vi "FGV ARN Test.vi"(7 "abgebrochen":bool, 10 "Aktion":T1=enum."init") -> (0 "Tabelle Wertänderung":bool, 1 "Fertig":bool, 2 "Aktion":T1=enum."init", 3 "Status":string)   [LabVIEW 2020, in "EPA 1065.lvlib" / "ARN Test 1065-305.lvlib"]
uses:
  ARN Test 1065-305.lvlib
  Aktion FGV ARN Test.ctl
  Aktion FGV ARN Daten.ctl
  Seiten/FT-IR/FGV FT-IR Aktionen.ctl
  Sprachverwaltung/FGV Aktion Tabelle zerlegen.ctl
  Seiten/CalGas Aufschaltung/FGV CalGas Aktionen.ctl
  Aktion FGV Graphen Daten.ctl
  Funktionstasten/Zustaende.ctl
  Funktionstasten/Funktionstasten-Aktion.ctl
  Seiten/CalGas Aufschaltung/Auswahl Aufschaltpunkt.ctl
  PNS/Aktionen FGV Grenzwerte.ctl
  Messdaten/Aktionen FGV Messdaten.ctl
  Messdaten/Gewichtung (Stichprobe).ctl
  Aktion FGV ARN Protokoll.ctl
  Funktionstasten/Funktionstasten.lvlib
  Messdaten/Messdaten.lvlib
  Seiten/FT-IR/FT-IR.lvlib
  Sprachverwaltung/Sprachverwaltung.lvlib
  Seiten/CalGas Aufschaltung/CalGas Aufschaltung.lvlib
  PNS/PNS.lvlib
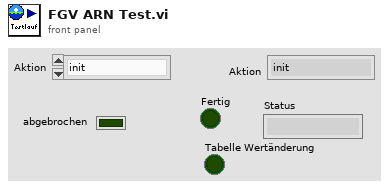
[diagram p1: front panel]
types:
  T1 = typedef "EPA 1065.lvlib/ARN Test 1065-305.lvlib/Aktion FGV ARN Test.ctl" = enum16{"leerlauf", "init", "lesen", "CG aufschalten", "Aufschaltzeit abwarten", "aufzeichnen vorbereiten", "aufzeichnen", "berechnen", "auswerten", "fertig", "0-Gas aufschalten", "0-Gas abwarten"}
  T2 = typedef "EPA 1065.lvlib/ARN Test 1065-305.lvlib/Aktion FGV Graphen Daten.ctl" = enum16{"init", "lesen", "Daten schreiben"}
  T3 = typedef "CalGas Aufschaltung.lvlib/FGV CalGas Aktionen.ctl" = enum16{"lesen", "Analysator Auswahl", "Def.CalGas", "Aufschaltung CalGas", "laden", "speichern", "KAL extrahieren"}
  T4 = enum16{"init", "lesen", "ARN Test aktiv", "ARN Test inaktiv"}
  T5 = typedef "Sprachverwaltung.lvlib/FGV Aktion Tabelle zerlegen.ctl" = enum16{"laden", "vereinzeln", "speichern"}
  T6 = typedef "EPA 1065.lvlib/ARN Test 1065-305.lvlib/Aktion FGV ARN Daten.ctl" = enum16{"Lesen", "laden", "speichern", "ARN Daten", "Rohdaten", "Rohdaten löschen", "Zeitstempel", "SNR Ergebnis"}
  T7 = typedef "FT-IR.lvlib/FGV FT-IR Aktionen.ctl" = enum16{"lesen", "NOG setzen", "NOS setzen", "Initialisieren", "speichern", "ALLES setzen", "FT-IR Spektrum loggen", "Komm Stoppen", "Spektrum LogKonfig"}
  T8 = typedef "Messdaten.lvlib/Aktionen FGV Messdaten.ctl" = enum16{"lesen", "schreiben", "löschen", "Mittelwerte", "Komponente"}
  T9 = typedef "CalGas Aufschaltung.lvlib/Auswahl Aufschaltpunkt.ctl" = enum16{"über Filterblock", "Analysator direkt", "über PNS", "Entnahme", "Gasdivider"}
  T10 = typedef "Funktionstasten.lvlib/Funktionstasten-Aktion.ctl" = enum16{"Initialisieren", "Zustand setzen", "Taste gedrückt", "Fehler speichern", "Lesen", "Manuell", "Remote", "Bitparallel", "Samplepoint", "Zeit Prüfen", "reset Umschalten"}
  T11 = typedef "Funktionstasten.lvlib/Zustaende.ctl" = enum16{"Standby", "Pause", "Eco", "Messen", "Kalibrieren", "Spülen Filter", "Spülen Leitung", "Umgebungsluft", "0-Gas", "Cal-Gas", "CG zu PNS", "-------------", "Init 1", "Init 2", "Init 3", "Init 4", "Messen vorbereiten", "Messen durchführen", "Exit"}
  T12 = typedef "PNS.lvlib/Aktionen FGV Grenzwerte.ctl" = enum16{"lesen", "Grenzw. schreiben", "Anweisungscode", "IP-Adresse", "laden", "speichern", "Anweisungscode vorgeben"}
  T13 = typedef "EPA 1065.lvlib/ARN Test 1065-305.lvlib/Aktion FGV ARN Protokoll.ctl" = enum16{"lesen", "Tab. schreiben", "Protokoll ausw.", "Protokoll speichern", "Textdatei speichern"}
  T14 = typedef "Messdaten.lvlib/Gewichtung (Stichprobe).ctl" = enum16{"Sample", "Population"}
  T15 = typedef "EPA 1065.lvlib/ARN Test 1065-305.lvlib/Allgemeine Einstellungen.ctl" = cluster{"Bearbeiter:":string, "Analysator":T16, "Komponente:":u16, "Gasflaschen Nr.:":string, "Accuracy":dbl, "Sollwert":dbl, "Modus":T17, "Pfad:":path, "Textname:":string, "CG Aufschaltzeit:":dbl, "Einheit":string, "N2 Aufschaltzeit:":dbl, "Gasflasche":T18, "Konfig Gasflasche":T19}
  T16 = typedef "System Einstellungen V2.lvlib/Analysatoren.ctl" = string
  T17 = typedef "EPA 1065.lvlib/T90 Test 1065-308.lvlib/Modus.ctl" = u16
  T18 = typedef "System Einstellungen V2.lvlib/Gasflasche Auswahl.ctl" = u16
  T19 = typedef "System Einstellungen V2.lvlib/Konfig Gasflasche.ctl" = bool
  T20 = typedef "CalGas Aufschaltung.lvlib/Aufschaltung CalGas.ctl" = cluster{"Kalibriergas":T21, "Aufschaltpunkt":T9, "Analysator":T22}
  T21 = typedef "Auswahlfeld.ctl" = u16
  T22 = typedef "CalGas Aufschaltung.lvlib/Auswahl Analysator.ctl" = enum16{"FT-IR", "FID", "PMA", "PMA/FID/FT-IR"}
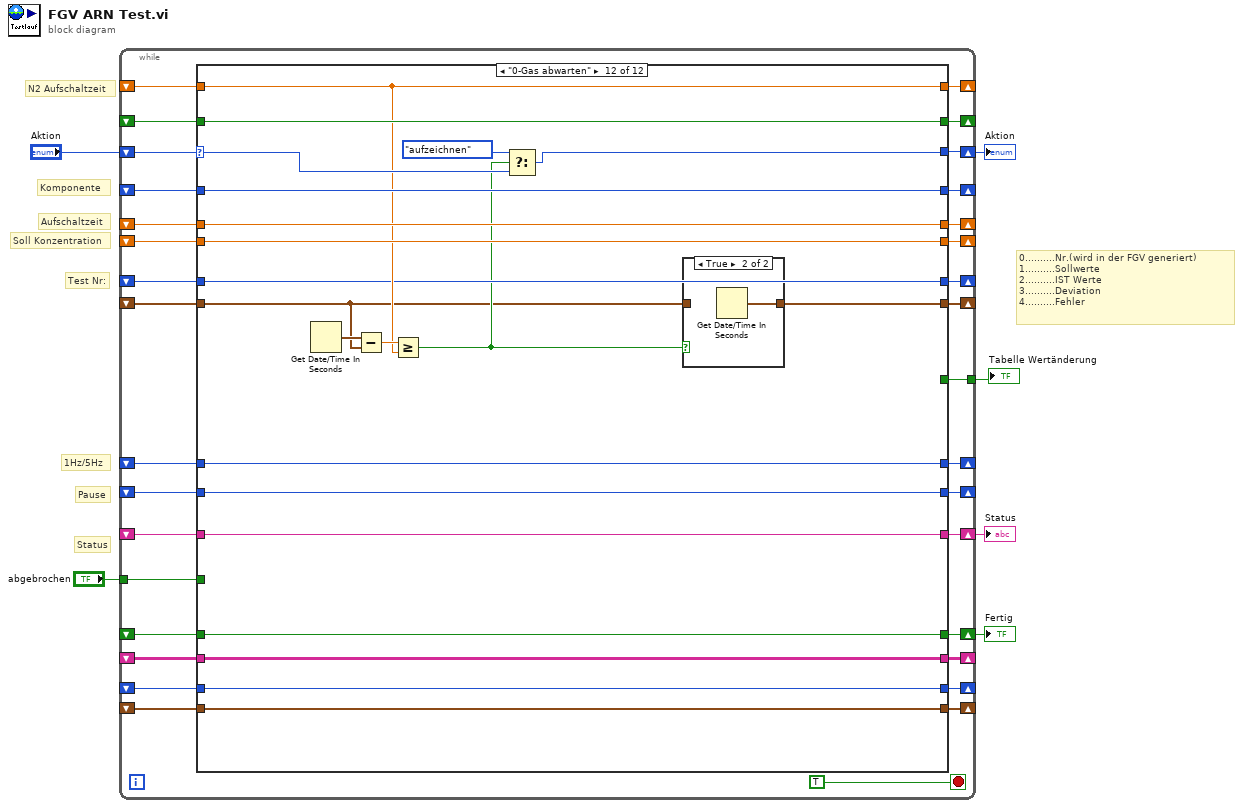
[diagram p0: block diagram]
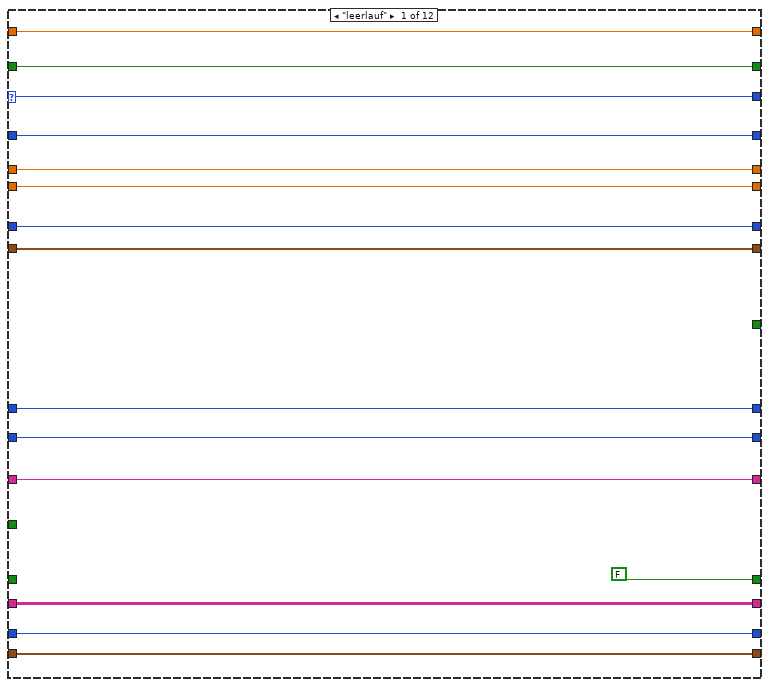
[diagram p2: hidden frame]
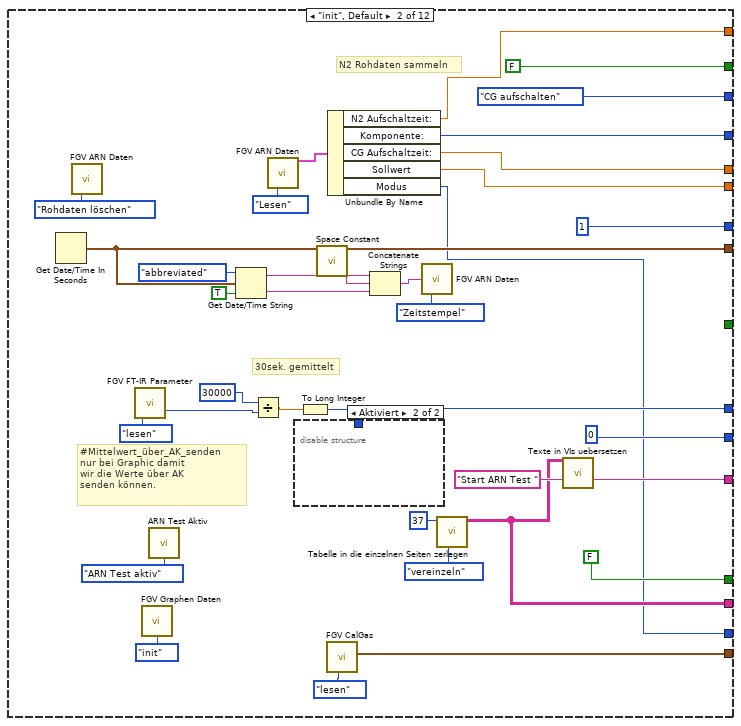
[diagram p3: hidden frame]
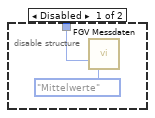
[diagram p4: hidden frame]
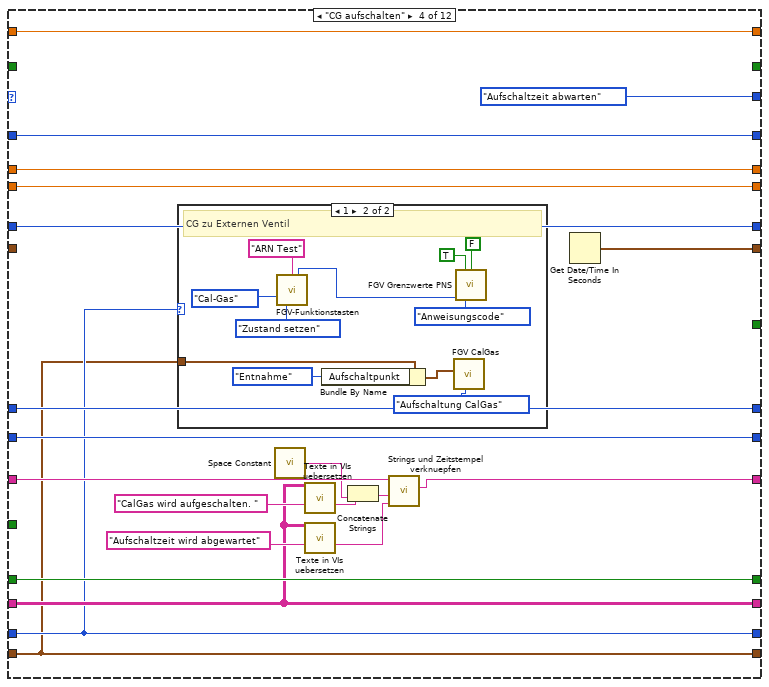
[diagram p6: hidden frame]
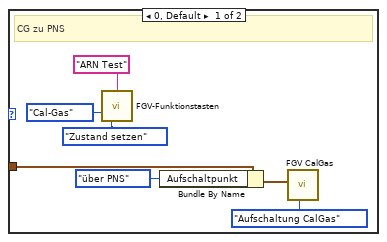
[diagram p7: hidden frame]
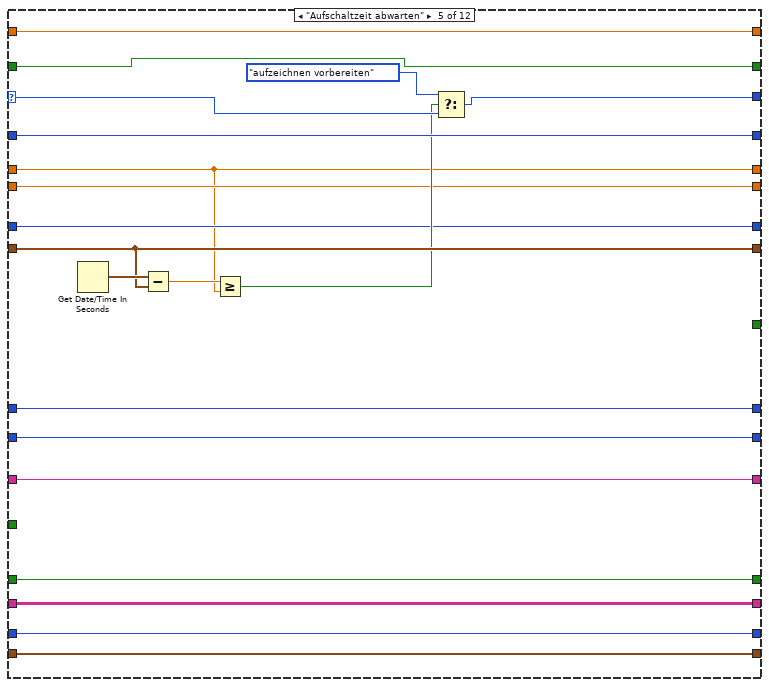
[diagram p8: hidden frame]
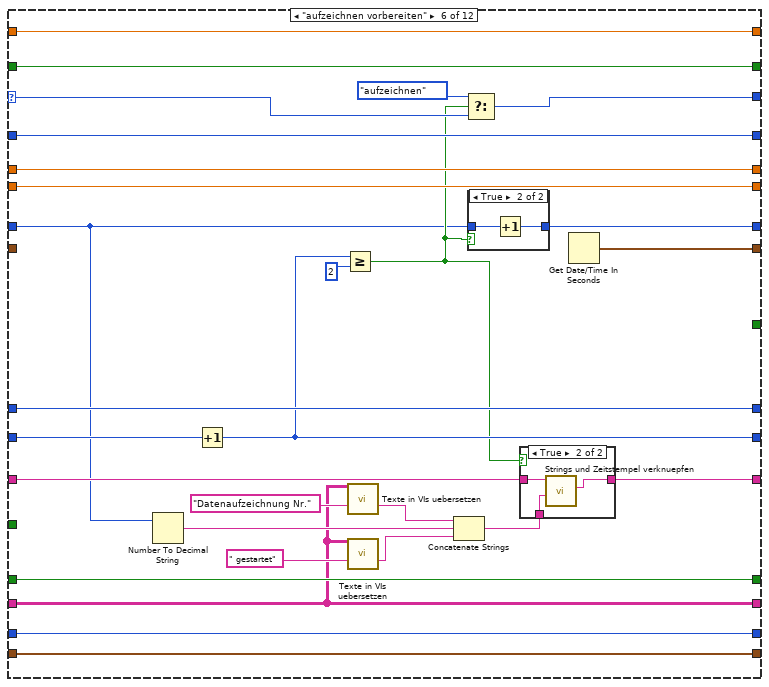
[diagram p9: hidden frame]
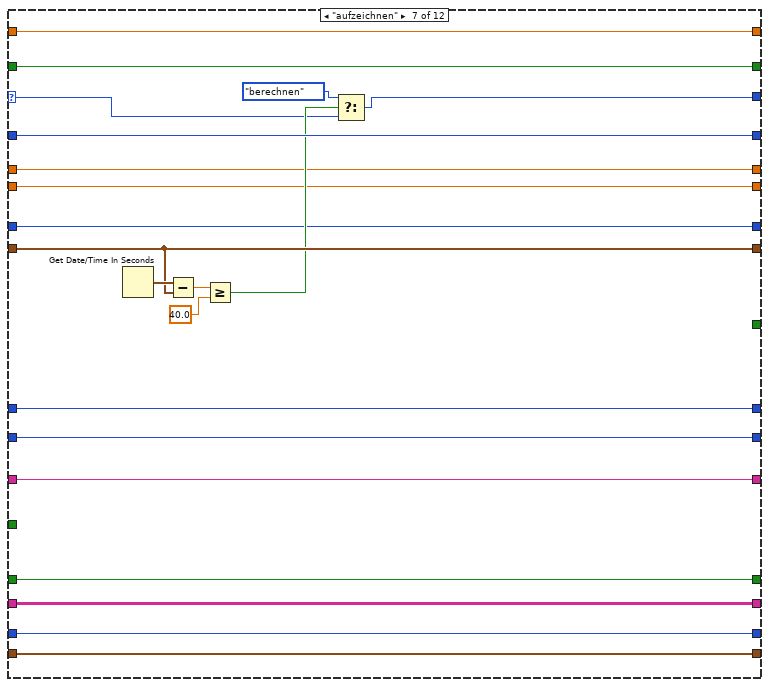
[diagram p12: hidden frame]
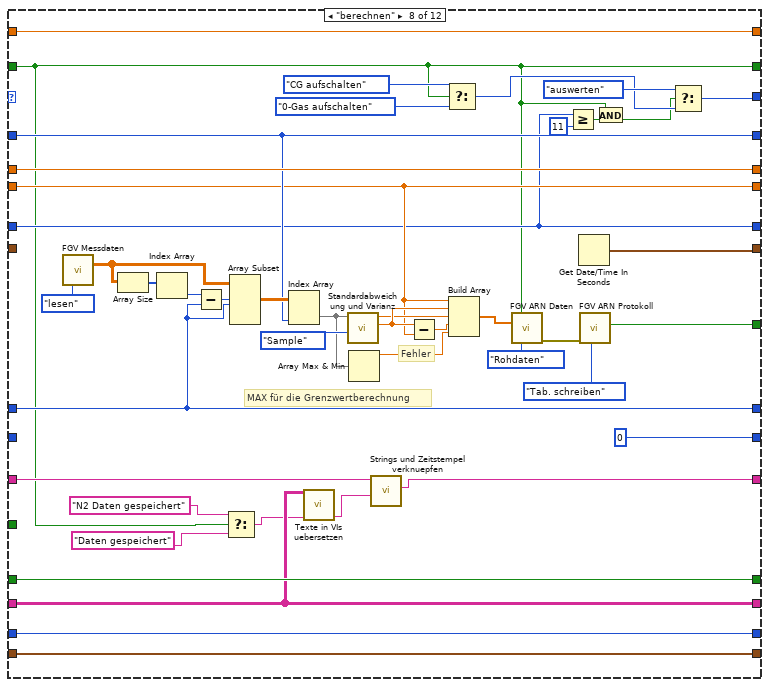
[diagram p13: hidden frame]
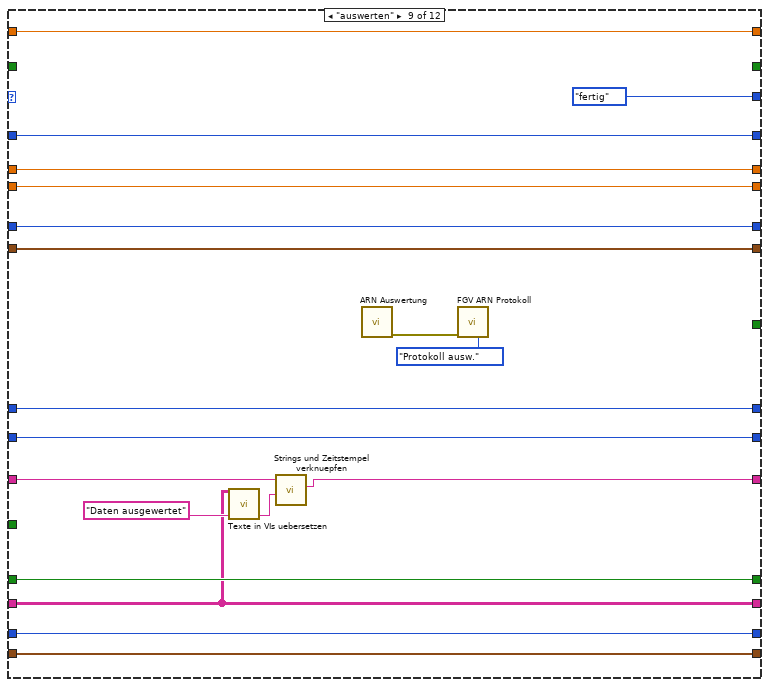
[diagram p14: hidden frame]
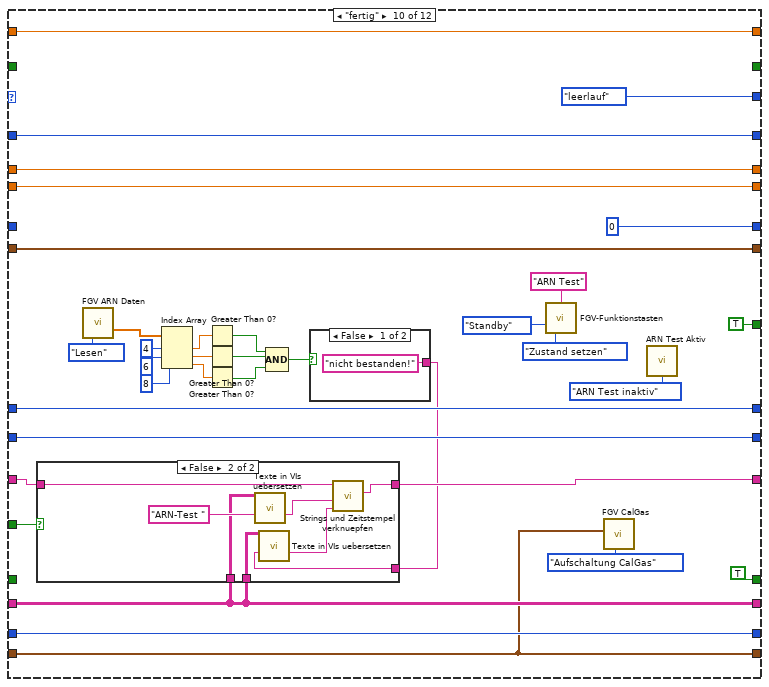
[diagram p15: hidden frame]
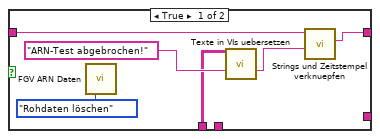
[diagram p16: hidden frame]
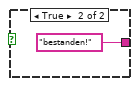
[diagram p17: hidden frame]
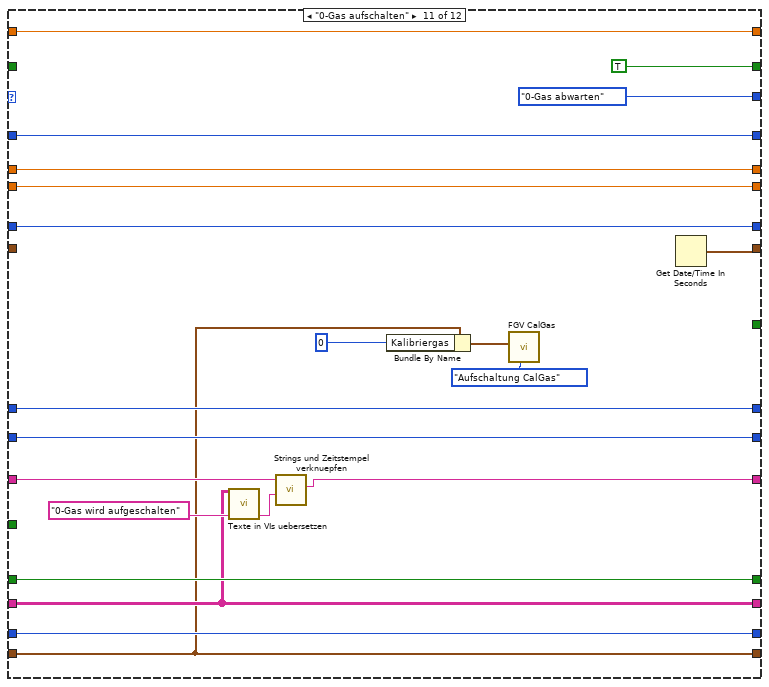
[diagram p18: hidden frame]
diagram:
  # "N2 Aufschaltzeit"
  # "0..........Nr.(wird in der FGV generiert)\n1..........Sollwerte\n2..........IST Werte\n3..........Deviation\n4..........Fehler"
  # "Status"
  # "1Hz/5Hz"
  # "Pause"
  # "Soll Konzentration"
  # "Test Nr:"
  # "Aufschaltzeit"
  # "Komponente"
  n1 = while {
    shift-right: [w37] -> _
    shift-left: _ -> [w36]
    shift-right: [w35] -> _
    shift-left: _ -> [w34]
    shift-right: [w33] -> _
    shift-left: _ -> [w32]
    shift-right: [w31] -> w5
    shift-left: "Aktion" -> [w38]
    shift-right: [w30] -> _
    shift-left: _ -> [w29]
    shift-right: [w28] -> _
    shift-left: _ -> [w27]
    shift-right: [w26] -> _
    shift-left: _ -> [w25]
    shift-right: [w24] -> _
    shift-left: _ -> [w23]
    shift-right: [w22] -> w4
    shift-left: _ -> [w21]
    tunnel: "abgebrochen" -> [w20]
    shift-right: [w19] -> w2
    shift-left: _ -> [w18]
    shift-right: [w17] -> _
    shift-left: _ -> [w16]
    shift-right: [w15] -> _
    shift-left: _ -> [w14]
    shift-right: [w13] -> _
    shift-left: _ -> [w12]
    shift-right: [w11] -> _
    shift-left: _ -> [w10]
    tunnel: [w9] -> w1
    shift-right: [w8] -> _
    shift-left: _ -> [w7]
    stop <- TRUE stop-if-true
    n2 = case shown="\"0-Gas abwarten\"" w38 {
      selector: w38 -> [w53 _ w102 _ w161 w185 w216 _ _ _ _ w363]
      tunnel: [w52 w87 w106 w127 w165 w193 w221 w257 w283 w319 w355 w377] -> w37
      tunnel: w36 -> [w52 _ w106 w127 w165 w193 w221 w257 w283 w319 w355 w377]
      tunnel: [w51 w86 w105 w126 w150 w192 w202 w265 w282 w318 w354 w376] -> w35
      tunnel: w34 -> [w51 _ w105 w126 w150 w192 w202 w265 w282 w318 w354 w376]
      tunnel: [w48 w78 w104 w125 w163 w191 w218 w239 w279 w316 w336 w358] -> w33
      tunnel: w32 -> [w48 _ w104 _ w163 _ w218 _ w279 w316 _ w357]
      tunnel: [w53 Aktion_FGV_ARN_Test."CG aufschalten" ("Aktion") w102 Aktion_FGV_ARN_Test."Aufschaltzeit abwarten" ("Aktion") w158 w184 w213 w225 Aktion_FGV_ARN_Test."fertig" ("Aktion") Aktion_FGV_ARN_Test."leerlauf" ("Aktion") Aktion_FGV_ARN_Test."0-Gas abwarten" ("Aktion") w361] -> w31
      tunnel: [w49 1 w103 w124 w157 w171 w211 w227 w280 0 w352 w360] -> w30
      tunnel: w29 -> [w49 _ w103 w124 w157 w170 w211 w227 w280 _ w352 w360]
      tunnel: [w50 w83 w101 w122 w156 w190 w214 w250 w281 w315 w353 w373] -> w28
      tunnel: w27 -> [w50 _ w101 w122 w156 w190 w214 w250 w281 w315 w353 w373]
      tunnel: [w47 w62 w100 w121 w155 w189 w212 w256 w278 w314 w351 w372] -> w26
      tunnel: w25 -> [w47 _ w100 w121 w155 w189 w212 w256 w278 w314 w351 w372]
      tunnel: [w46 0 w99 w120 w154 w183 w210 0 w277 w313 w350 w371] -> w24
      tunnel: w23 -> [w46 _ w99 w120 w154 w188 w210 _ w277 w313 w350 w371]
      tunnel: [w45 w68 w98 w118 w153 w180 w209 w246 w275 w311 w348 w370] -> w22
      tunnel: w21 -> [w45 _ w98 w119 w153 w181 w209 w247 w276 w312 w349 w370]
      tunnel: w20 -> [_ _ _ _ _ _ _ _ _ w297 _ _]
      tunnel: [FALSE ("abgebrochen") FALSE ("abgebrochen") w97 w117 w152 w178 w208 w242 w272 TRUE ("abgebrochen") w347 w369] -> w19
      tunnel: w18 -> [_ _ w97 w117 w152 w178 w208 w242 w272 _ w347 w369]
      tunnel: [w44 w67 w96 w113 w151 w173 w207 w240 w269 w292 w344 w368] -> w17
      tunnel: w16 -> [w44 _ w96 w113 w151 w173 w207 w240 w269 w292 w344 w368]
      tunnel: [w54 FALSE w95 _ w149 w169 w206 w222 _ _ TRUE w366] -> w15
      tunnel: w14 -> [w54 _ w95 _ w149 w169 w206 w222 _ _ _ w366]
      tunnel: [w42 w58 w94 w108 w148 w168 w205 w233 w268 w287 w339 w365] -> w13
      tunnel: w12 -> [w42 _ w94 w108 w148 w168 w205 w233 w268 w287 w339 w365]
      tunnel: [w41 w57 w93 w109 w147 w167 w204 w232 w267 w289 w342 w364] -> w11
      tunnel: w10 -> [w41 _ w93 w109 w147 w167 w204 w232 w267 w289 w342 w364]
      tunnel: [_ _ _ _ _ _ _ w231 _ TRUE ("Tabelle Wertänderung") _ _] -> w9
      tunnel: [w40 w55 w92 w107 w146 w166 w203 w230 w266 w285 w337 w362] -> w8
      tunnel: w7 -> [w40 _ w92 w107 w146 w166 w203 w230 w266 w285 w337 w362]
      frame "leerlauf" {
      }
      frame "init", Default {
        # "#Mittelwert_über_AK_senden\nnur bei Graphic damit\nwir die Werte über AK \nsenden können."
        # "N2 Rohdaten sammeln"
        # "30sek. gemittelt"
        n3 = Get Date/Time In Seconds() -> (seconds since 1Jan1904=w78:timestamp)
        n4 = call "FGV ARN Daten.vi"("Aktion"=Aktion_FGV_ARN_Daten."Rohdaten löschen") -> ()  [unwired: 9 in, 6 out]
        n5 = call "FGV FT-IR Parameter.vi"("Aktion"=FGV_FT-IR_Aktionen."lesen") -> ("Zykluszeit Messdatenverteiler"=w64:u32)  [unwired: 11 in, 7 out]
        n6 = call "FGV Graphen Daten.vi"("Aktion"=Aktion_FGV_Graphen_Daten."init") -> ()  [unwired: 12 in, 3 out]
        n7 = call "ARN Test Aktiv.vi"("Aktion"=T4."ARN Test aktiv") -> ()  [unwired: 13 in, 2 out]
        n8 = Get Date/Time String(date format (0)=enum16{"short", "long", "abbreviated"}."abbreviated" ("Datumsformat (0)"), seconds (now)=w78, want seconds? (F)=TRUE ("Angabe von Sekunden? (F)")) -> (date string=w75:string, time string=w73:string)
        n9 = Divide(x=30000, y=w64) -> (x/y=w63:dbl)
        n10 = call "FGV ARN Daten.vi"("Aktion"=Aktion_FGV_ARN_Daten."Lesen") -> ("ARN Konfig Daten"=w88:T15)  [unwired: 9 in, 5 out]
        n11 = To Long Integer(number=w63) -> (32bit integer=w62:i32)
        n12 = disable-structure shown="Aktiviert" {
          disable-tunnel: w62 -> [w90 _]
          frame Disabled {
            n13 = call "FGV Messdaten.vi"("Mittelwerte"=w90, "Aktionen"=Aktionen_FGV_Messdaten."Mittelwerte") -> ()  [unwired: 5 in, 9 out]
          }
          frame Enabled {
          }
        }
        n14 = call <vilib>:"Space Constant.vi"() -> ("String"=w74:string)
        n15 = call "FGV CalGas.vi"("Aktionen"=FGV_CalGas_Aktionen."lesen") -> ("Aufschaltung CalGas"=w58:T20)  [unwired: 6 in, 4 out]
        n16 = Unbundle By Name(w88) -> ("N2 Aufschaltzeit:"=w55:dbl, "Komponente:"=w87:u16, "CG Aufschaltzeit:"=w86:dbl, "Sollwert"=w83:dbl, "Modus"=w57:T17)
        n17 = Concatenate Strings(w75, w74, w73) -> (w72:string)
        n18 = call "FGV ARN Daten.vi"("Zeitstempel"=w72, "Aktion"=Aktion_FGV_ARN_Daten."Zeitstempel") -> ()  [unwired: 8 in, 6 out]
        n19 = call "Tabelle in die einzelnen Seiten zerlegen.vi"("Aktion"=FGV_Aktion_Tabelle_zerlegen."vereinzeln", "Index (Seite)"=37) -> ("Sprachliste"=w67:string[][])  [unwired: 7 in, 2 out]
        n20 = call "Texte in VIs uebersetzen.vi"("Sprachliste"=w67, "String zum Übersetzen"="Start ARN Test ") -> ("String zum Übersetzen"=w68:string)  [unwired: 9 in, 4 out]
      }
      frame "lesen" {
      }
      frame "CG aufschalten" {
        n21 = case shown="1" w109 {
          tunnel: w108 -> [w130 w137]
          frame 0, Default {
            # "CG zu PNS"
            n22 = call "FGV-Funktionstasten.vi"("Herkunft"="ARN Test", "Zustand"=Zustaende."Cal-Gas", "Aktion"=Funktionstasten-Aktion."Zustand setzen") -> ()  [unwired: 5 in, 8 out]
            n23 = Bundle By Name(cluster=w130, "Aufschaltpunkt"=Auswahl_Aufschaltpunkt."über PNS") -> (w128:T20)
            n24 = call "FGV CalGas.vi"("Aktionen"=FGV_CalGas_Aktionen."Aufschaltung CalGas", "Aufschaltung CalGas"=w128) -> ()  [unwired: 5 in, 5 out]
          }
          frame 1 {
            # "CG zu Externen Ventil"
            n25 = call "FGV-Funktionstasten.vi"("Herkunft"="ARN Test", "Zustand"=Zustaende."Cal-Gas", "Aktion"=Funktionstasten-Aktion."Zustand setzen") -> ("Samplepoint"=w139:u16)  [unwired: 5 in, 7 out]
            n26 = Bundle By Name(cluster=w137, "Aufschaltpunkt"=Auswahl_Aufschaltpunkt."Entnahme") -> (w136:T20)
            n27 = call "FGV CalGas.vi"("Aktionen"=FGV_CalGas_Aktionen."Aufschaltung CalGas", "Aufschaltung CalGas"=w136) -> ()  [unwired: 5 in, 5 out]
            n28 = call "FGV Grenzwerte PNS.vi"("T90"=TRUE ("T90 lüften"), "T90 lüften"=FALSE, "Samplepoint"=w139, "Aktionen FGV Grenzwerte"=Aktionen_FGV_Grenzwerte."Anweisungscode") -> ()  [unwired: 9 in, 3 out]
          }
        }
        n29 = call <vilib>:"Space Constant.vi"() -> ("String"=w111:string)
        n30 = call "Texte in VIs uebersetzen.vi"("Sprachliste"=w113, "String zum Übersetzen"="CalGas wird aufgeschalten. " ("String 1 hinzufügen")) -> ("String zum Übersetzen"=w112:string)  [unwired: 9 in, 4 out]
        n31 = call "Texte in VIs uebersetzen.vi"("Sprachliste"=w113, "String zum Übersetzen"="Aufschaltzeit wird abgewartet" ("String 2 hinzufügen")) -> ("String zum Übersetzen"=w115:string)  [unwired: 9 in, 4 out]
        n32 = Concatenate Strings(w112, w111) -> (w110:string)
        n33 = call "Strings und Zeitstempel verknuepfen.vi"("String 2 hinzufügen"=w115, "String 1 hinzufügen"=w110, "Eingagns String"=w119) -> ("Verknüpfter String"=w118:string)  [unwired: 8 in]
        n34 = Get Date/Time In Seconds() -> (seconds since 1Jan1904=w125:timestamp)
      }
      frame "Aufschaltzeit abwarten" {
        n35 = Get Date/Time In Seconds() -> (seconds since 1Jan1904=w164:timestamp)
        n36 = Subtract(x=w164, y=w163) -> (x-y=w162:dbl)
        n37 = Greater Or Equal?(x=w162, y=w150) -> (x >= y?=w160:bool)
        n38 = Select(t=Aktion_FGV_ARN_Test."aufzeichnen vorbereiten", s=w160, f=w161) -> (s? t:f=w158:T1)
      }
      frame "aufzeichnen vorbereiten" {
        n39 = Number To Decimal String(number=w170) -> (decimal integer string=w182:string)  [unwired: 1 in]
        n40 = Increment(x=w188) -> (x+1=w183:i32)
        n41 = Greater Or Equal?(x=w183, y=2) -> (x >= y?=w172:bool)
        n42 = call "Texte in VIs uebersetzen.vi"("Sprachliste"=w173, "String zum Übersetzen"="Datenaufzeichnung Nr." ("String")) -> ("String zum Übersetzen"=w176:string)  [unwired: 9 in, 4 out]
        n43 = call "Texte in VIs uebersetzen.vi"("Sprachliste"=w173, "String zum Übersetzen"=" gestartet" ("String")) -> ("String zum Übersetzen"=w174:string)  [unwired: 9 in, 4 out]
        n44 = Concatenate Strings(w176, w182, w174) -> (w179:string)
        n45 = Select(t=Aktion_FGV_ARN_Test."aufzeichnen" ("Aktion"), s=w172, f=w185) -> (s? t:f=w184:T1)
        n46 = case shown="True" w172 {
          tunnel: [w194 w195] -> w171
          tunnel: w170 -> [w194 w196]
          frame False {
          }
          frame True {
            n47 = Increment(x=w196) -> (x+1=w195:i32)
          }
        }
        n48 = case shown="True" w172 {
          tunnel: w181 -> [w197 w200]
          tunnel: [w197 w198] -> w180
          tunnel: w179 -> [_ w199]
          frame False {
          }
          frame True {
            n49 = call "Strings und Zeitstempel verknuepfen.vi"("String 1 hinzufügen"=w199, "Eingagns String"=w200) -> ("Verknüpfter String"=w198:string)  [unwired: 9 in]
          }
        }
        n50 = Get Date/Time In Seconds() -> (seconds since 1Jan1904=w191:timestamp)
      }
      frame "aufzeichnen" {
        n51 = Get Date/Time In Seconds() -> (seconds since 1Jan1904=w219:timestamp)
        n52 = Subtract(x=w219, y=w218) -> (x-y=w220:dbl)
        n53 = Greater Or Equal?(x=w220, y=40.0) -> (x >= y?=w217:bool)
        n54 = Select(t=Aktion_FGV_ARN_Test."berechnen" ("Aktion"), s=w217, f=w216) -> (s? t:f=w213:T1)
      }
      frame "berechnen" {
        # "MAX für die Grenzwertberechnung"
        # "Fehler"
        n55 = call "FGV Messdaten.vi"("Aktionen"=Aktionen_FGV_Messdaten."lesen") -> ("Messdaten"=w260:sgl[][])  [unwired: 6 in, 8 out]
        n56 = Array Size(array=w260) -> (size(s)=w263:i32[])
        n57 = Index Array(array=w263) -> (element=w262:i32)  [unwired: 1 in]
        n58 = Subtract(x=w262, y=w256) -> (x-y=w261:i32)
        n59 = Select(t="N2 Daten gespeichert" ("String 1 hinzufügen"), s=w222, f="Daten gespeichert" ("String 1 hinzufügen")) -> (s? t:f=w236:string)
        n60 = Array Subset(array=w260, index (row)=w261, length (row)=w256) -> (w258:sgl[][])  [unwired: 2 in]
        n61 = Index Array(array=w258, index (col)=w257) -> (element=w249:sgl[])  [unwired: 1 in]
        n62 = call "Texte in VIs uebersetzen.vi"("Sprachliste"=w240, "String zum Übersetzen"=w236) -> ("String zum Übersetzen"=w241:string)  [unwired: 9 in, 4 out]
        n63 = call "Standardabweichung und Varianz.vi"("Gewichtung (Stichprobe)"=Gewichtung_(Stichprobe)."Sample", "X"=w249) -> ("Mittelwert"=w255:sgl, "Standardabweichung"=w254:sgl)  [unwired: 7 in, 1 out]
        n64 = Array Max & Min(array=w249) -> (max value=w248:sgl)  [unwired: 3 out]
        n65 = call "Strings und Zeitstempel verknuepfen.vi"("String 1 hinzufügen"=w241, "Eingagns String"=w247) -> ("Verknüpfter String"=w246:string)  [unwired: 9 in]
        n66 = Subtract(x=w255, y=w250) -> (x-y=w253:dbl)
        n67 = Select(t=Aktion_FGV_ARN_Test."CG aufschalten" ("Aktion"), s=w222, f=Aktion_FGV_ARN_Test."0-Gas aufschalten" ("Aktion")) -> (s? t:f=w224:T1)
        n68 = Build Array(w250, w255, w254, w253, w248) -> (w252:dbl[])
        n69 = call "FGV ARN Daten.vi"("N2"=w222, "Rohdaten"=w252, "Aktion"=Aktion_FGV_ARN_Daten."Rohdaten") -> ("error out"=w243:errorcluster)  [unwired: 7 in, 5 out]
        n70 = Greater Or Equal?(x=w227, y=11) -> (x >= y?=w226:bool)
        n71 = Get Date/Time In Seconds() -> (seconds since 1Jan1904=w239:timestamp)
        n72 = call "FGV ARN Protokoll.vi"("Aktion"=Aktion_FGV_ARN_Protokoll."Tab. schreiben", "error in (no error)"=w243) -> ("Tabelle Wertänderung"=w231:bool)  [unwired: 7 in, 2 out]
        n73 = And(x=w222, y=w226) -> (x .and. y?=w223:bool)
        n74 = Select(t=Aktion_FGV_ARN_Test."auswerten" ("Aktion"), s=w223, f=w224) -> (s? t:f=w225:T1)
      }
      frame "auswerten" {
        n75 = call "Texte in VIs uebersetzen.vi"("Sprachliste"=w269, "String zum Übersetzen"="Daten ausgewertet" ("String 1 hinzufügen")) -> ("String zum Übersetzen"=w271:string)  [unwired: 9 in, 4 out]
        n76 = call "Strings und Zeitstempel verknuepfen.vi"("String 1 hinzufügen"=w271, "Eingagns String"=w276) -> ("Verknüpfter String"=w275:string)  [unwired: 9 in]
        n77 = call "ARN Auswertung.vi"() -> ("error out"=w273:errorcluster)  [unwired: 11 in]
        n78 = call "FGV ARN Protokoll.vi"("Aktion"=Aktion_FGV_ARN_Protokoll."Protokoll ausw.", "error in (no error)"=w273) -> ()  [unwired: 7 in, 3 out]
      }
      frame "fertig" {
        n79 = call "FGV ARN Daten.vi"("Aktion"=Aktion_FGV_ARN_Daten."Lesen") -> ("SNR Ergebnis"=w309:sgl[])  [unwired: 9 in, 5 out]
        n80 = Index Array(array=w309, index #1=4 ("Index"), index #2=6 ("Index"), index #3=8 ("Index")) -> (element #1=w301:sgl, element #2=w300:sgl, element #3=w299:sgl)
        n81 = Greater Than 0?(x=w301) -> (x > 0?=w305:bool)
        n82 = Greater Than 0?(x=w300) -> (x > 0?=w303:bool)
        n83 = Greater Than 0?(x=w299) -> (x > 0?=w302:bool)
        n84 = Compound Arithmetic op=AND ("Mehrfacharithmetik")(w305, w303, w302) -> (w304:bool)
        n85 = case shown="False" w304 {
          tunnel: ["nicht bestanden!" "bestanden!"] -> w298
          frame False {
          }
          frame True {
          }
        }
        n86 = case shown="False" w297 {
          tunnel: w312 -> [w325 w333]
          tunnel: [w324 w332] -> w311
          tunnel: w298 -> [_ w328]
          tunnel: w292 -> [w320 w329]
          tunnel: w292 -> [_ w326]
          frame True {
            n87 = call "FGV ARN Daten.vi"("Aktion"=Aktion_FGV_ARN_Daten."Rohdaten löschen") -> ()  [unwired: 9 in, 6 out]
            n88 = call "Texte in VIs uebersetzen.vi"("Sprachliste"=w320, "String zum Übersetzen"="ARN-Test abgebrochen!" ("String 1 hinzufügen")) -> ("String zum Übersetzen"=w321:string)  [unwired: 9 in, 4 out]
            n89 = call "Strings und Zeitstempel verknuepfen.vi"("String 1 hinzufügen"=w321, "Eingagns String"=w325) -> ("Verknüpfter String"=w324:string)  [unwired: 9 in]
          }
          frame False {
            n90 = call "Texte in VIs uebersetzen.vi"("Sprachliste"=w329, "String zum Übersetzen"="ARN-Test " ("String 1 hinzufügen")) -> ("String zum Übersetzen"=w330:string)  [unwired: 9 in, 4 out]
            n91 = call "Texte in VIs uebersetzen.vi"("Sprachliste"=w326, "String zum Übersetzen"=w328) -> ("String zum Übersetzen"=w327:string)  [unwired: 9 in, 4 out]
            n92 = call "Strings und Zeitstempel verknuepfen.vi"("String 2 hinzufügen"=w327, "String 1 hinzufügen"=w330, "Eingagns String"=w333) -> ("Verknüpfter String"=w332:string)  [unwired: 8 in]
          }
        }
        n93 = call "FGV-Funktionstasten.vi"("Herkunft"="ARN Test", "Zustand"=Zustaende."Standby", "Aktion"=Funktionstasten-Aktion."Zustand setzen") -> ()  [unwired: 5 in, 8 out]
        n94 = call "FGV CalGas.vi"("Aktionen"=FGV_CalGas_Aktionen."Aufschaltung CalGas", "Aufschaltung CalGas"=w287) -> ()  [unwired: 5 in, 5 out]
        n95 = call "ARN Test Aktiv.vi"("Aktion"=T4."ARN Test inaktiv") -> ()  [unwired: 13 in, 2 out]
      }
      frame "0-Gas aufschalten" {
        n96 = call "Texte in VIs uebersetzen.vi"("Sprachliste"=w344, "String zum Übersetzen"="0-Gas wird aufgeschalten" ("String 1 hinzufügen")) -> ("String zum Übersetzen"=w346:string)  [unwired: 9 in, 4 out]
        n97 = call "Strings und Zeitstempel verknuepfen.vi"("String 1 hinzufügen"=w346, "Eingagns String"=w349) -> ("Verknüpfter String"=w348:string)  [unwired: 9 in]
        n98 = Bundle By Name(cluster=w339, "Kalibriergas"=0) -> (w340:T20)
        n99 = call "FGV CalGas.vi"("Aktionen"=FGV_CalGas_Aktionen."Aufschaltung CalGas", "Aufschaltung CalGas"=w340) -> ()  [unwired: 5 in, 5 out]
        n100 = Get Date/Time In Seconds() -> (seconds since 1Jan1904=w336:timestamp)
      }
      frame "0-Gas abwarten" {
        n101 = Get Date/Time In Seconds() -> (seconds since 1Jan1904=w374:timestamp)
        n102 = Subtract(x=w374, y=w357) -> (x-y=w375:dbl)
        n103 = Greater Or Equal?(x=w375, y=w362) -> (x >= y?=w359:bool)
        n104 = Select(t=Aktion_FGV_ARN_Test."aufzeichnen" ("Aktion"), s=w359, f=w363) -> (s? t:f=w361:T1)
        n105 = case shown="True" w359 {
          tunnel: [w378 w379] -> w358
          tunnel: w357 -> [w378 _]
          frame False {
          }
          frame True {
            n106 = Get Date/Time In Seconds() -> (seconds since 1Jan1904=w379:timestamp)
          }
        }
      }
    }
  }
  "Aktion" <- w5
  "Status" <- w4
  "Fertig" <- w2
  "Tabelle Wertänderung" <- w1
